vi "Reset Generator.vi"(0 "RedPitaya connection in":refnum<k5>, 5 "error in":errorcluster, 12 "timeout ms (2000)":i32=2000) -> (14 "RedPitaya connection out":refnum<k5>, 19 "error out":errorcluster)   [LabVIEW 2010, in "RedPitaya.lvlib"]
doc: "Reset generator to default settings"
uses:
  RedPitaya.lvlib
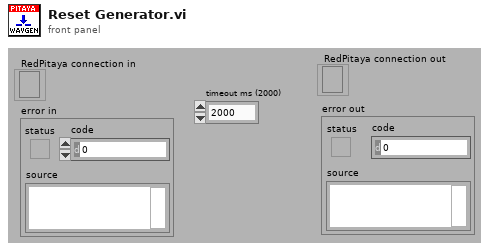
[diagram p1: front panel]
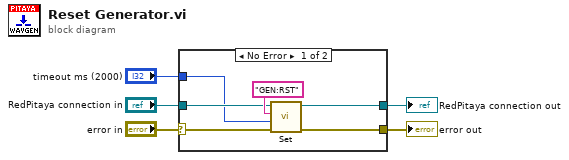
[diagram p0: block diagram]
diagram:
  n1 = case shown="No Error" "error in" {
    selector: "error in" -> [w7 w13]
    tunnel: "RedPitaya connection in" -> [w10 w12]
    tunnel: [w9 w13] -> w4
    tunnel: [w8 w12] -> w3
    tunnel: "timeout ms (2000)" -> [w6 _]
    frame No Error {
      n2 = call "Set.vi"("error in"=w7, "timeout ms (2000)"=w6, "SCPI Message"="GEN:RST", "RedPitaya connection in"=w10) -> ("error out"=w9:errorcluster, "RedPitaya connection out"=w8:refnum<k5>)  [unwired: 5 in, 1 out]
    }
    frame Error {
    }
  }
  "error out" <- w4
  "RedPitaya connection out" <- w3
